vi "PicoScope6000ExampleBlock.vi"() -> ()   [LabVIEW 2010]
uses:
  shared/PicoBuffers.ctl
  shared/Buffer and Transfer Settings.ctl
  shared/Acquisition Settings.ctl
  PicoScope6000Lib/PicoScope6000AnalogChannelSettings.ctl
panel:
  in  "Trigger Settings":T1={"Trigger Enabled"=FALSE, "Trigger Source"=enum."Channel A", "Trigger Threshold (Volts)"=0.0, "Trigger Direction"=2, "Trigger Delay (samples)"=0, "Auto Trigger Time (ms)"=1000} {"Trigger Direction" items=["Rising"=2, "Falling"=3]}
  in  "Write to File":bool
  in  "Channel B Settings":T2={"Enabled"=FALSE, "Coupling"=1, "Range"=6, "Analogue Offset"=0.0, "Bandwidth"=0} {"Bandwidth" items=["Full", "20 MHz"]; "Range" items=["10 mV", "20 mV", "50 mV", "100 mV", "200 mV", "500 mV", "1 V", "2 V", "5 V", "10 V", "20 V", "50 V ", "100 V"]; "Coupling" items=["AC", "DC 1 MOhm", "DC 50 Ohm"]}
  out "Device Info":T3
  out "Properties Panel":T4 {"Max Total Capture Time Available (sec)" format="%.3p"; "Sample Frequency" format="%.3p"; "Sample Internal" format="%.3p"; "Max Samples Available" format="%.3p"; "Total Capture Time (sec)" format="%.3p"}
  in  "Channel A Settings":T2={"Enabled"=TRUE, "Coupling"=1, "Range"=6, "Analogue Offset"=0.0, "Bandwidth"=0} {"Bandwidth" items=["Full", "20 MHz"]; "Range" items=["10 mV", "20 mV", "50 mV", "100 mV", "200 mV", "500 mV", "1 V", "2 V", "5 V", "10 V", "20 V", "50 V ", "100 V"]; "Coupling" items=["AC", "DC 1 MOhm", "DC 50 Ohm"]}
  out "Pico 6000 Units":string
  out "error out":errorcluster
  in  "Data file":path=path "PicoScope6000ExampleBlock ChA Data"
  in  "Acquisition Settings":T5={"preTriggerSamples"=0, "postTriggerSamples"=5000000, "timebase"=5} {"postTriggerSamples" format="%_6p"; "preTriggerSamples" format="%_6p"}
  in  "Buffer and Transfer Settings":T6={"startIndex"=0, "Samples"=5000000, "Down Sample Ratio"=1, "Down-Sample Mode"=0} {"Down-Sample Mode" items=["RAW none"=2147483648, "None"=0, "Aggregate"=1, "Decimate"=2, "Average"=4]; "Down Sample Ratio" step=1; "Samples" format="%_6p"}
  in  "stop":bool
  out "Analog Channels":cluster{i32, sgl, "Data":dbl[]}[](graph)
  in  "Apply Settings":bool
  out "overflow":i16 format="%04b"
  in  "Serial Number":string
  in  "Use Serial Number":bool
  in  "error in (no error)":errorcluster
  # "Bit 0 = ChA"
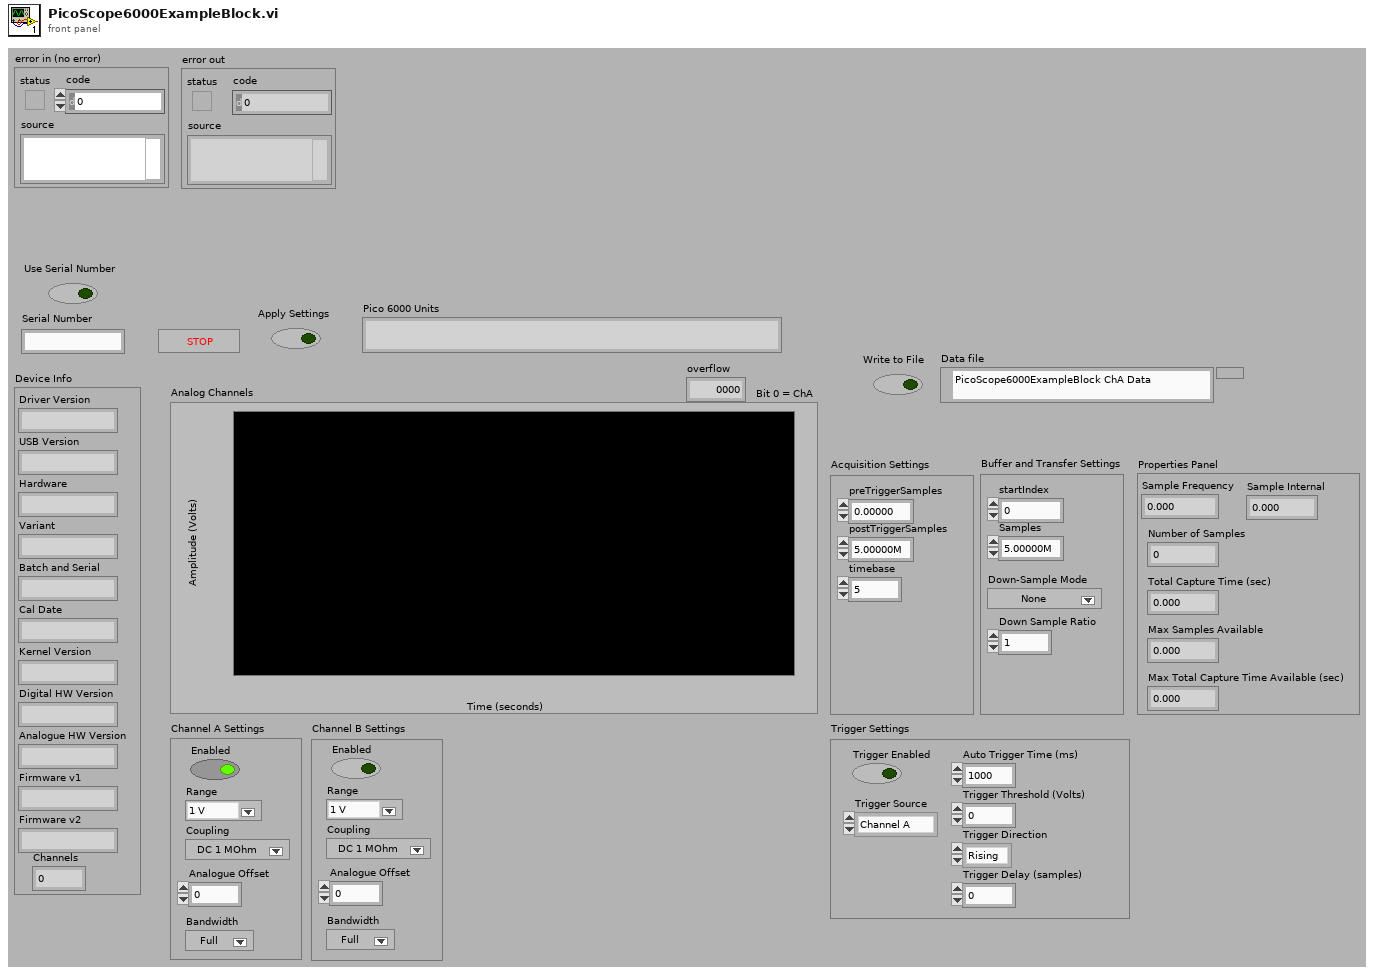
[diagram p1: front panel]
types:
  T1 = cluster{"Trigger Enabled":bool, "Trigger Source":enum32{"Channel A", "Channel B", "Channel C", "Channel D", "External", "Aux."}, "Trigger Threshold (Volts)":dbl, "Trigger Direction":u16, "Trigger Delay (samples)":u32, "Auto Trigger Time (ms)":i16}
  T2 = typedef "PicoScope6000AnalogChannelSettings.ctl" = cluster{"Enabled":bool, "Coupling":u32, "Range":u32, "Analogue Offset":sgl, "Bandwidth":u32}
  T3 = cluster{"Driver Version":string, "USB Version":string, "Hardware":string, "Variant":string, "Batch and Serial":string, "Cal Date":string, "Kernel Version":string, "Digital HW Version":string, "Analogue HW Version":string, "Firmware v1":string, "Firmware v2":string, "Channels":i16}
  T4 = cluster{"Sample Frequency":sgl, "Sample Internal":sgl, "maxSamples":u32, "Number of Samples":u32, "Total Capture Time (sec) ":sgl, "Max Total Capture Time Available (sec)":sgl}
  T5 = typedef "Acquisition Settings.ctl" = cluster{"preTriggerSamples":u64, "postTriggerSamples":u64, "timebase":u32}
  T6 = typedef "Buffer and Transfer Settings.ctl" = cluster{"startIndex":u64, "Samples":u64, "Down Sample Ratio":u64, "Down-Sample Mode":u32}
  T7 = typedef "PicoBuffers.ctl" = cluster{"Max Buffer Pointers":u64[][][], "Min Buffer Pointers":u64[][][], "StreamingDataInfo":cluster{"Channel":u32, "Down-Sample Mode":u32, "PICO_DATA_TYPE":enum32{"PICO_INT8_T", "PICO_INT16_T", "PICO_INT32_T", "PICO_UINT32_T", "PICO_INT64_T", ""}, "Samples":i32, "bufferIndex":u64, "startIndex":i32, "overflow":i16}[][]}
  T8 = enum16{"open", "open or create", "create or replace", "create", "open (read-only)"}
  T9 = cluster{"Channel A Buffer":i16[], "Channel B Buffer":i16[], "Channel C Buffer":i16[], "Channel D Buffer":i16[], "Channel E Buffer":i16[], "Channel F Buffer":i16[], "Channel G Buffer":i16[], "Channel H Buffer":i16[], "Port 0 Buffer":i16[], "Port 1 Buffer":i16[]}[]
  T10 = cluster{"Channel A Buffer":i16[], "Channel B Buffer":i16[], "Channel C Buffer":i16[], "Channel D Buffer":i16[], "Channel E Buffer":i16[], "Channel F Buffer":i16[], "Channel G Buffer":i16[], "Channel H Buffer":i16[], "Port 0 Buffer":i16[], "Port 1 Buffer":i16[]}
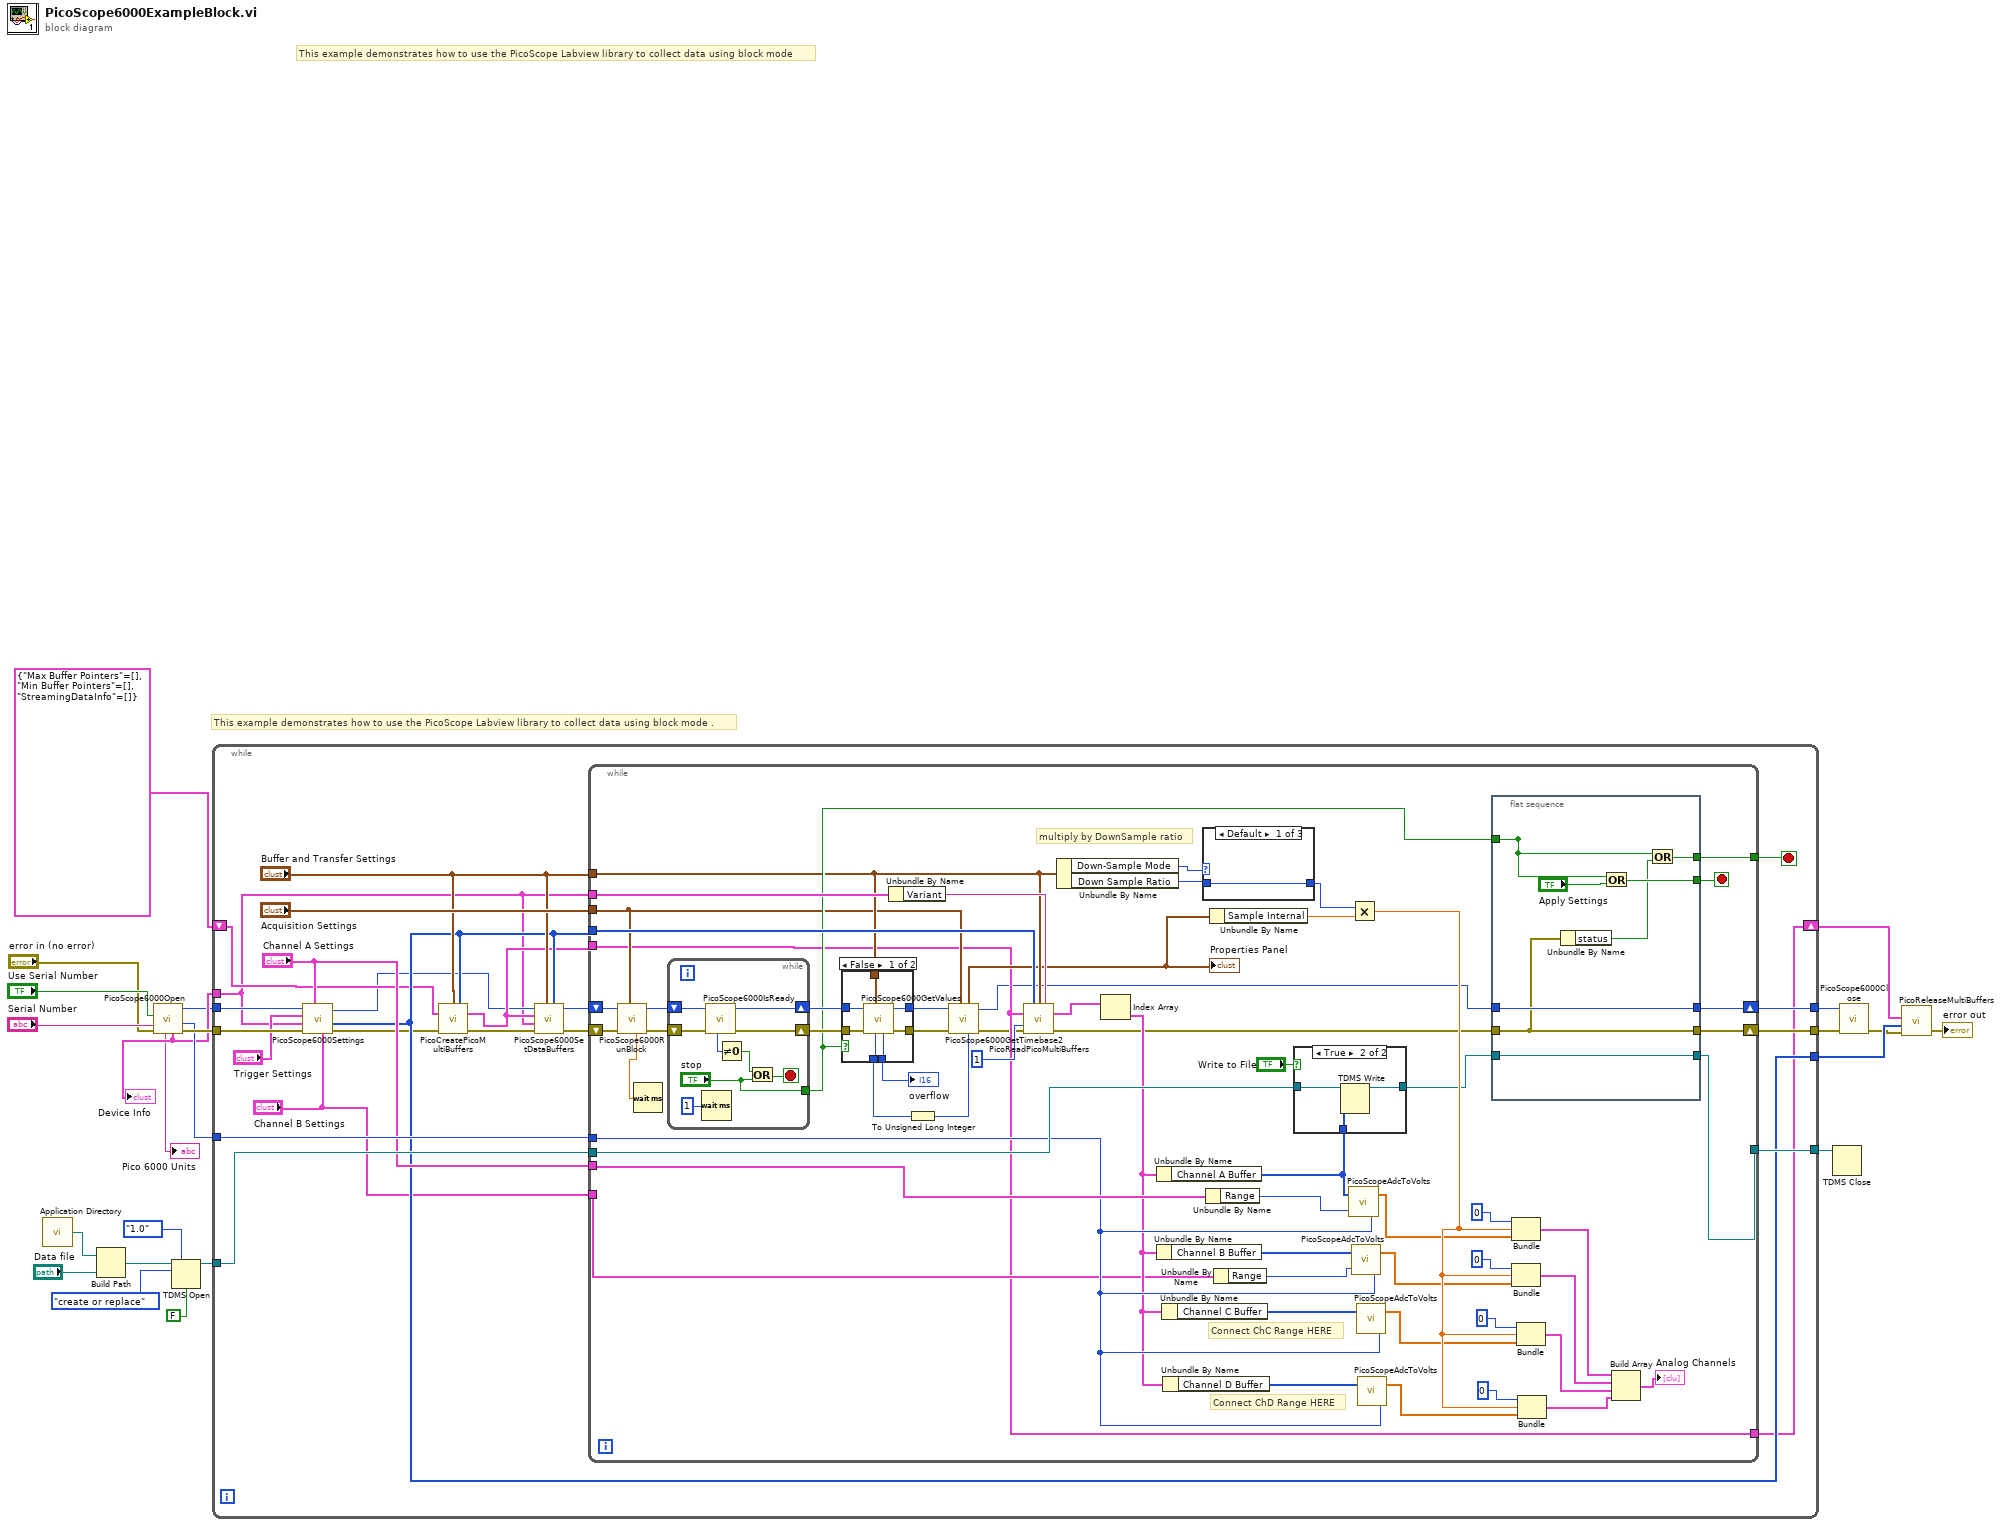
[diagram p0: block diagram]
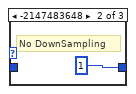
[diagram p4: hidden frame]
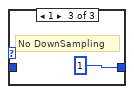
[diagram p5: hidden frame]
diagram:
  # "This example demonstrates how to use the PicoScope Labview library to collect data using block mode ."
  # "This example demonstrates how to use the PicoScope Labview library to collect data using block mode"
  n1 = call <vilib>:"Application Directory.vi"() -> ("Application Directory"=w16:path)
  n2 = Build Path(base path=w16, name or relative path="Data file") -> (appended path=w17:path)
  n3 = call "PicoScope6000Open.vi"("error in (no error)"="error in (no error)", "Serial Number"="Serial Number", "Use Serial Number"="Use Serial Number") -> ("error out"=w9:errorcluster, "Max Adc value"=w7:i16, "handle"=w1:i16, "Device Info"=w6:T3, "Pico 6000 Units"=→"Pico 6000 Units":string)  [unwired: 4 in]
  "Device Info" <- w6
  n4 = TDMS Open(6:FALSE ("disable buffering? (T)"), 7:enum16{"1.0", "2.0"}."1.0" ("file format version (2.0)"), 10:T8."create or replace" ("operation (0:open)"), 11:w17) -> (3:w14:refnum<k34>)  [unwired: 2 in, 1 out]
  n5 = while {
    tunnel: w7 -> [w40]
    tunnel: [w34] -> w23
    tunnel: [w43] -> w15
    tunnel: w14 -> [w46]
    tunnel: w6 -> [w24]
    tunnel: w9 -> [w28]
    tunnel: [w44] -> w3
    tunnel: [w41] -> w12
    shift-right: [w31] -> w22
    shift-left: T7 {"Max Buffer Pointers"=[], "Min Buffer Pointers"=[], "StreamingDataInfo"=[]} ("Data Pointers") -> [w30]
    tunnel: w1 -> [w27]
    stop <- w42 stop-if-true
    n6 = call "PicoScope6000Settings.vi"("Channel B Settings"="Channel B Settings", "Channel A Settings"="Channel A Settings", "error in"=w28, "Device Info"=w24, "Trigger Settings"="Trigger Settings", "handle in"=w27) -> ("error out"=w29:errorcluster, "Enabled array"=w34:i16[], "handle out"=w26:i16)  [unwired: 3 in]
    n7 = call "PicoCreatePicoMultiBuffers.vi"("Buffer and Transfer Settings"="Buffer and Transfer Settings", "enabled array"=w34, "Data Pointers In"=w30, "error in (no error)"=w29) -> ("Data Pointers"=w33:T7, "error out"=w37:errorcluster)  [unwired: 10 in]
    n8 = call "PicoScope6000SetDataBuffers.vi"("enabled array"=w34, "Buffer and Transfer Settings"="Buffer and Transfer Settings", "error in (no error)"=w37, "Device Info"=w24, "Data Pointers In"=w33, "handle in"=w26) -> ("error out"=w39:errorcluster, "handle out"=w38:i16)  [unwired: 4 in]
    n9 = while {
      tunnel: w33 -> [w52]
      tunnel: "Buffer and Transfer Settings" -> [w63]
      tunnel: w34 -> [w101]
      tunnel: "Channel A Settings" -> [w100]
      tunnel: "Acquisition Settings" -> [w56]
      tunnel: w40 -> [w99]
      tunnel: w24 -> [w96]
      tunnel: [w71] -> w42
      shift-right: [w75] -> w44
      shift-left: w39 -> [w61]
      shift-right: [w69] -> w41
      shift-left: w38 -> [w62]
      tunnel: w46 -> [w107]
      tunnel: [w73] -> w43
      tunnel: "Channel B Settings" -> [w53]
      tunnel: [w52] -> w31
      stop <- w70 stop-if-true
      # "Connect ChD Range HERE"
      # "Connect ChC Range HERE"
      # "multiply by DownSample ratio"
      n10 = call "PicoScope6000RunBlock.vi"("Acquisition Settings"=w56, "error in (no error)"=w61, "handle in"=w62) -> ("error out"=w60:errorcluster, "handle out"=w59:i16, "timeIndisposedMs"=w58:dbl)  [unwired: 5 in, 1 out]
      n11 = Wait (ms)(milliseconds to wait=w58) -> ()  [unwired: 1 out]
      n12 = while {
        shift-right: [w130] -> w67
        shift-left: w60 -> [w134]
        shift-right: [w131] -> w68
        shift-left: w59 -> [w133]
        tunnel: ["stop"] -> w66
        stop <- w136 stop-if-true
        n13 = Wait (ms)(milliseconds to wait=u32 1) -> ()  [unwired: 1 out]
        n14 = call "PicoScope6000IsReady.vi"("error in (no error)"=w134, "handle in"=w133) -> ("error out"=w130:errorcluster, "handle out"=w131:i16, "ready"=w129:i16)  [unwired: 7 in]
        n15 = Not Equal To 0?(x=w129) -> (x != 0?=w137:bool)
        n16 = Or(x=w137, y="stop") -> (x .or. y?=w136:bool)
      }
      n17 = case shown="False" w66 {
        tunnel: w67 -> [w117 w119]
        tunnel: w68 -> [w116 w120]
        tunnel: [w115 w120] -> w49
        tunnel: [w118 w119] -> w50
        tunnel: w63 -> [w114 _]
        tunnel: [w113 _] -> w65
        tunnel: [w112 _] -> w64
        frame False {
          n18 = call "PicoScope6000GetValues.vi"("Buffer and Transfer Settings"=w114, "error in (no error)"=w117, "handle in"=w116) -> ("error out"=w118:errorcluster, "handle out"=w115:i16, "overflow"=w113:i16, "noOfSamples"=w112:u64)  [unwired: 5 in]
        }
        frame True {
        }
      }
      "overflow" <- w65
      n19 = Unbundle By Name(w96) -> ("Variant"=w97:string)
      n20 = To Unsigned Long Integer(number=w64) -> (unsigned 32bit integer=w57:u32)
      n21 = call "PicoScope6000GetTimebase2.vi"("Number of Samples"=w57, "Acquisition Settings"=w56, "error in (no error)"=w50, "handle in"=w49) -> ("error out"=w48:errorcluster, "handle out"=w47:i16, "Properties Panel"=w55:T4)  [unwired: 5 in]
      "Properties Panel" <- w55
      n22 = call "PicoReadPicoMultiBuffers.vi"("enabled array"=w101, "Buffer and Transfer Settings"=w63, "Variant"=w97, "Data Pointers"=w52, "No of Buffers"=1, "error in (no error)"=w48) -> ("MultiBuffers (Max or non-aggregated)"=w106:T9, "error out"=w72:errorcluster)  [unwired: 7 in, 1 out]
      n23 = Unbundle By Name(w63) -> ("Down-Sample Mode"=w104:u32, "Down Sample Ratio"=w105:u64)
      n24 = Index Array(array=w106) -> (element=w76:T10)  [unwired: 1 in]
      n25 = Unbundle By Name(w76) -> ("Channel A Buffer"=w85:i16[])
      n26 = Unbundle By Name(w76) -> ("Channel B Buffer"=w91:i16[])
      n27 = Unbundle By Name(w76) -> ("Channel C Buffer"=w83:i16[])
      n28 = Unbundle By Name(w76) -> ("Channel D Buffer"=w79:i16[])
      n29 = case shown="Default" w104 {
        tunnel: [w138 u64 1 ("Down Sample Ratio") u64 1 ("Down Sample Ratio")] -> w102
        tunnel: w105 -> [w138 _ _]
        frame Default {
        }
        frame -2147483648 {
          # "No DownSampling"
        }
        frame 1 {
          # "No DownSampling"
        }
      }
      n30 = Unbundle By Name(w100) -> ("Range"=w93:u32)
      n31 = Unbundle By Name(w55) -> ("Sample Internal"=w98:sgl)
      n32 = Unbundle By Name(w53) -> ("Range"=w54:u32)
      n33 = case shown="True" "Write to File" {
        tunnel: w107 -> [w108 w111]
        tunnel: w85 -> [_ w110]
        tunnel: [w108 w109] -> w74
        frame False {
        }
        frame True {
          n34 = TDMS Write(0:w111, 9:w110) -> (4:w109:refnum<k34>)  [unwired: 4 in, 3 out]
        }
      }
      n35 = call "PicoScopeAdcToVolts.vi"("Max_adc"=w99, "Range Index"=w93, "Data"=w85) -> ("Data"=w86:dbl[])
      n36 = Multiply(x=w102, y=w98) -> (x*y=w103:sgl)
      n37 = call "PicoScopeAdcToVolts.vi"("Max_adc"=w99, "Range Index"=w54, "Data"=w91) -> ("Data"=w90:dbl[])
      n38 = call "PicoScopeAdcToVolts.vi"("Max_adc"=w99, "Data"=w83) -> ("Data"=w82:dbl[])  [unwired: 1 in]
      n39 = call "PicoScopeAdcToVolts.vi"("Max_adc"=w99, "Data"=w79) -> ("Data"=w78:dbl[])  [unwired: 1 in]
      n40 = flat-sequence {
        tunnel: [w128] -> w70
        tunnel: [w121] -> _
        tunnel: [w125] -> w71
        tunnel: w47 -> [w124]
        tunnel: [w124] -> w69
        tunnel: w72 -> [w123]
        tunnel: [w123] -> w75
        tunnel: [w122] -> w73
        tunnel: w74 -> [w122]
        tunnel: w66 -> [w121]
        frame #0 {
          n41 = Unbundle By Name(w123) -> ("status"=w126:bool)
          n42 = Or(x=w121, y="Apply Settings") -> (x .or. y?=w128:bool)
          n43 = Or(x=w121, y=w126) -> (x .or. y?=w125:bool)
        }
      }
      n44 = Bundle(0, w103, "Data"=w86) -> (w89:cluster{i32, sgl, "Data":dbl[]})  [unwired: 1 in]
      n45 = Bundle(0, w103, "Data"=w90) -> (w88:cluster{i32, sgl, "Data":dbl[]})  [unwired: 1 in]
      n46 = Bundle(0, w103, "Data"=w82) -> (w81:cluster{i32, sgl, "Data":dbl[]})  [unwired: 1 in]
      n47 = Bundle(0, w103, "Data"=w78) -> (w77:cluster{i32, sgl, "Data":dbl[]})  [unwired: 1 in]
      n48 = Build Array(w89, w88, w81, w77) -> (→"Analog Channels":cluster{i32, sgl, "Data":dbl[]}[])
    }
  }
  n49 = TDMS Close(11:w15) -> ()  [unwired: 1 in, 2 out]
  n50 = call "PicoScope6000Close.vi"("error in (no error)"=w3, "handle"=w12) -> ("error out"=w2:errorcluster)  [unwired: 8 in, 1 out]
  n51 = call "PicoReleaseMultiBuffers.vi"("error in (no error)"=w2, "Enabled array"=w23, "Data Pointers"=w22) -> ("error out"=→"error out":errorcluster)  [unwired: 7 in, 1 out]
